vi "Find Index of Timestamps.vi"(10 "System Time (s)":dbl[](array[numeric]), 11 "Test TimeStamps (us)":i64[](array[numeric])) -> (3 "Test TDMS Offsets":i64[](array[numeric]))   [LabVIEW 2011]
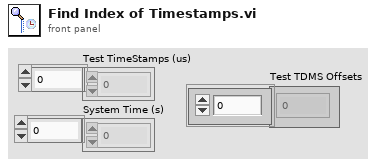
[diagram p1: front panel]
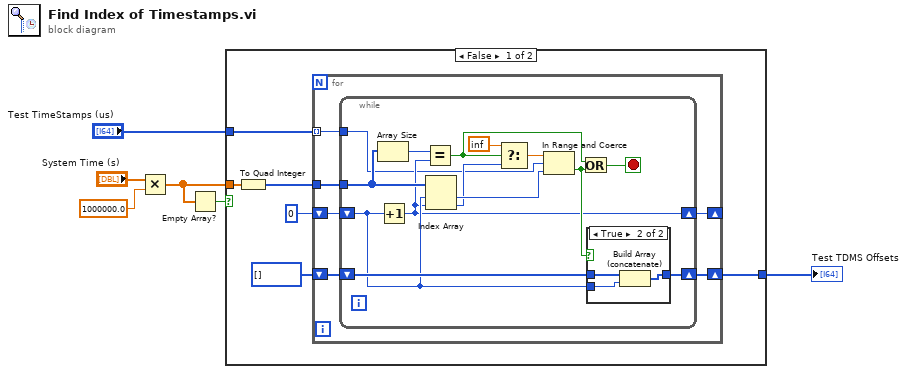
[diagram p0: block diagram]
diagram:
  n1 = Multiply(x="System Time (s)", y=1000000.0) -> (x*y=w2:dbl[])
  n2 = Empty Array?(array=w2) -> (empty?=w1:bool)
  n3 = case shown="False" w1 {
    tunnel: w2 -> [w12 _]
    tunnel: [w10 _] -> w4
    tunnel: "Test TimeStamps (us)" -> [w8 _]
    frame False {
      n4 = To Quad Integer(1:w12) -> (0:w7:i64[])
      n5 = for {
        tunnel: w8 -> [w17] mode=indexing
        tunnel: w7 -> [w18]
        shift-right: [w15] -> w10
        shift-left: i64[] [] -> [w16]
        shift-right: [w13] -> _
        shift-left: i64 0 -> [w14]
        n6 = while {
          tunnel: w18 -> [w27]
          shift-right: [w25] -> w13
          shift-left: w14 -> [w29]
          tunnel: w17 -> [w19]
          shift-right: [w30] -> w15
          shift-left: w16 -> [w31]
          stop <- w21 stop-if-true
          n7 = Array Size(array=w27) -> (size(s)=w26:i32)
          n8 = Increment(x=w29) -> (x+1=w25:i64)
          n9 = Equal?(x=w26, y=w25) -> (x = y?=w20:bool)
          n10 = Index Array(array=w27, index #1=w29, index #2=w25) -> (element #1=w32:i64, element #2=w24:i64)
          n11 = Select(t=inf, s=w20, f=w24) -> (s? t:f=w23:dbl)
          n12 = In Range and Coerce(upper limit=w23, x=w19, lower limit=w32) -> (In Range?=w28:bool)  [unwired: 1 out]
          n13 = Or(x=w20, y=w28) -> (x .or. y?=w21:bool)
          n14 = case shown="True" w28 {
            tunnel: w31 -> [w33 w36]
            tunnel: [w33 w34] -> w30
            tunnel: w29 -> [_ w35]
            frame False {
            }
            frame True {
              n15 = Build Array (concatenate)(w36, w35) -> (w34:i64[])
            }
          }
        }
      }
    }
    frame True {
    }
  }
  "Test TDMS Offsets" <- w4
